vi "Export Multirate FIR Coefficients to Xilinx COE File.vi"() -> ()   [LabVIEW 2023]
doc: "Demonstrates how to export integer finite impulse response (FIR) coefficients of a multirate filter from a text file that you generated using the DFD Save MRate to Text File VI. This example also demonstrates how to use the exported coefficients to build a .coe file. To create the .coe file, specify a valid path to the .coe file in the <B>COE File Path</B> input. You can load the .coe filter using the Xilinx CORE Generator (TM).\n\nXilinx (R) is the registered trademark of Xilinx, Inc."
uses:
  <vilib>/addons/Digital Filter Design/_Objects.llb/DFD Coef Norm Type.ctl
  <vilib>/addons/Digital Filter Design/FilterLib.llb/DFD Save MRate Filter to Text File.vi
  <vilib>/addons/Digital Filter Design/NI_DigFilterLicensed.lvlib
panel:
  in  "Coefficient Type":T1(ring)
  out "Error Message":string
  in  "COE File Path":path
  out "COE Text":string
  in  "Text Filter File Path":path
  in  "Coefficients Word Length":i16=16
  # "Select Help>>Show Context Help and move the cursor over the VI icon for more information."
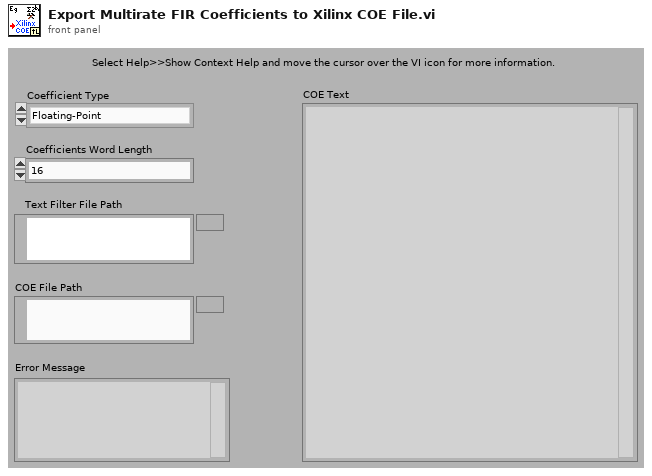
[diagram p1: front panel]
types:
  T1 = enum16{"Floating-Point", "Fixed-Point", "Integer"}
  T2 = typedef "NI_DigFilterLicensed.lvlib/DFD Coef Norm Type.ctl" = enum16{"No Norm", "Time Domain 1-Norm", "Time Domain 2-Norm", "Time Domain Inf-Norm"}
  T3 = typedef "NI_DigFilterLicensed.lvlib/DFD Multirate Filter Obj.ctl" = cluster{"mMRate_Structure":enum16{"CIC", "FIR", "IIR", "Lattice"}, "mMRate_Mode":T4, "mMRate_Factor":i32, "mMRate_FIRParams":cluster{"mMRate_FIR_H":dbl[], "mMRate_FIR_IsNyquist?":bool, "mMRate_FIR_IsSymmetric?":bool}, "mMRate_CICParams":cluster{"mMRate_CIC_#Stage":i32, "mMRate_CIC_Lag":i32, "mMRate_CIC_Type":enum16{"Lowpass", "Highpass"}}, "mMRate_Order":i32, "mMRate_Version":string, "mMRate_Comments":string, "mMRate_RationalFactor":cluster{"mMRate_L":i32, "mMRate_M":i32}, "mMRate_Fs":dbl, "mMRate_Quantized?":bool, "mMRate_QFilterGain":dbl, "mMRate_CoefWl":i16, "mMRate_Scaling":cluster{"mMRate_ScaleByPowerOf2?":bool, "mMRate_ScaleType":T2}, "mMRate_InputWl":i16, "mMRate_OutputWl":i16, "mMRate_OutputMode":T5, "mMRate_MultMode":T6, "mMRate_BitPruning":bool, "mMRate_GainWl":i16, "mMRate_OutputFwl":i16, "mMRate_SumIwl":i16, "mMRate_InputIwl ":i16, "mMRate_SumWl":i16, "mMRate_CoefIwl":i16}
  T4 = typedef "NI_DigFilterLicensed.lvlib/DFD Multirate Mode.ctl" = i16
  T5 = typedef "NI_DigFilterLicensed.lvlib/DFD Round-off Mode.ctl" = enum16{"Nearest", "Truncation"}
  T6 = typedef "NI_DigFilterLicensed.lvlib/DFD FXP MRate Multiply Mode.ctl" = enum16{"Truncated", "Full"}
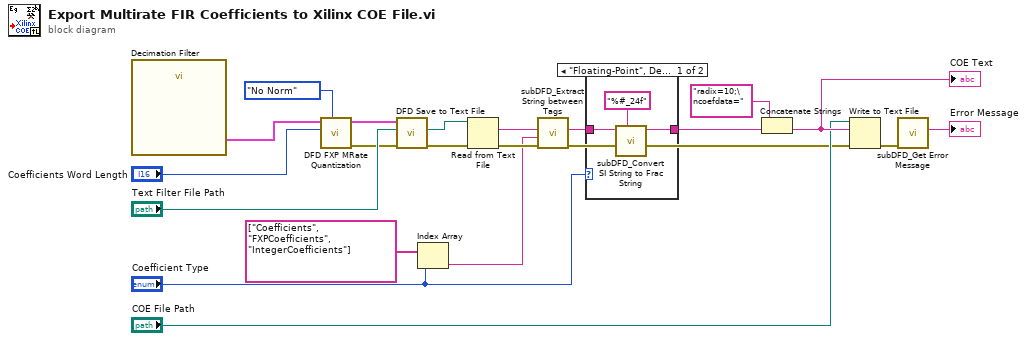
[diagram p0: block diagram]
diagram:
  n1 = call "Decimation Filter"() -> ("multirate filter out"=w6:T3)  [unwired: 11 out]
  n2 = call <vilib>:"DFD FXP MRate Quantization.vi"("scale type"=DFD_Coef_Norm_Type."No Norm", "coefficients word length"="Coefficients Word Length", "multirate filter in"=w6) -> ("error out"=w17:errorcluster, "multirate filter out"=w19:T3)  [unwired: 3 in, 4 out]
  n3 = call-poly <vilib>:"DFD Save to Text File.vi"("error in (no error)"=w17, "file path in"="Text Filter File Path", "multirate filter in"=w19) -> ("error out"=w15:errorcluster, "file path out"=w16:path)  [unwired: 1 in, 6 out]
  n4 = Index Array(array=string[] ["Coefficients", "FXPCoefficients", "IntegerCoefficients"], index="Coefficient Type") -> (element=w4:string)
  n5 = Read from Text File(file (use dialog)=w16, error in=w15) -> (text=w14:string, error out=w10:errorcluster)  [unwired: 4 out]
  n6 = call "subDFD_Extract String between Tags.vi"("tag"=w4, "original string"=w14) -> ("extracted string"=w2:string)  [unwired: 1 in, 8 out]
  n7 = case shown="\"Floating-Point\", Default" "Coefficient Type" {
    tunnel: w2 -> [w22 w24]
    tunnel: [w21 w24] -> w1
    frame "Floating-Point", Default {
      n8 = call "subDFD_Convert SI String to Frac String.vi"("format string"="%#_24f", "SI string in"=w22) -> ("Fractional string out"=w21:string)  [unwired: 9 out]
    }
    frame "Integer" {
    }
  }
  n9 = Concatenate Strings("radix=10;\ncoefdata=", w1) -> (w12:string)
  "COE Text" <- w12
  n10 = Write to Text File(file (use dialog)="COE File Path", text=w12, error in=w10) -> (error out=w9:errorcluster)  [unwired: 3 out]
  n11 = call <vilib>:"subDFD_Get Error Message.vi"("error in (no error)"=w9) -> ("Error Message"=→"Error Message":string)  [unwired: 10 out]
